vi "Invalid Text Color Write.vi"(4 "error in (no error)":errorcluster, 5 "Value":u32(colorbox)=8388608, 6 "Container State":T2, 7 "Display State In":T1={"format string"="%#_g", "font size"=13, "invalid text"="<Auto>", "valid range"={"min"=-inf, "max"=0.0}, "size"={"width"=100, "height"=22}, "numeric text color"=0, "overlay text color"=6553600}) -> (0 "error out":errorcluster, 3 "Display State Out":T1={"format string"="%#_g", "font size"=13, "invalid text"="<Auto>", "valid range"={"min"=-inf, "max"=0.0}, "size"={"width"=100, "height"=22}, "numeric text color"=0, "overlay text color"=6553600})   [LabVIEW 2017, in "Numeric with String Overlay.xctl"]
uses:
  <vilib>/addons/_XControls/Numeric with String Overlay/Numeric with String Overlay.xctl
  <vilib>/_xctls/Container State.ctl
  <vilib>/addons/_XControls/Numeric with String Overlay/State.ctl
  <vilib>/_xctls/XControlSupport.lvlib
panel:
  # "Replace the Value Control below with a Control of desired type.\nDo not remove this Control or the others from the connector pane.\nDo not change the connector pane pattern.\nThe Value control should always be the third terminal from top on the input side in the connector pane."
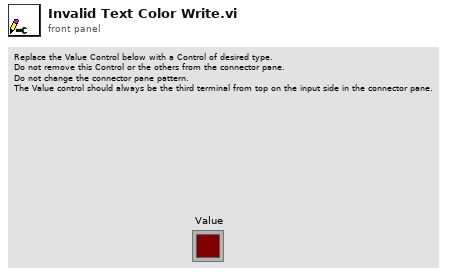
[diagram p1: front panel]
types:
  T1 = typedef "Numeric with String Overlay.xctl/State.ctl" = cluster{"format string":string, "font size":u32, "invalid text":string, "valid range":cluster{"min":dbl, "max":dbl}, "size":cluster{"width":u32, "height":u32}, "numeric text color":u32, "overlay text color":u32}
  T2 = typedef "XControlSupport.lvlib/Container State.ctl" = cluster{"Indicator?":bool, "Run Mode?":bool, " Refnum":refnum<vi>}
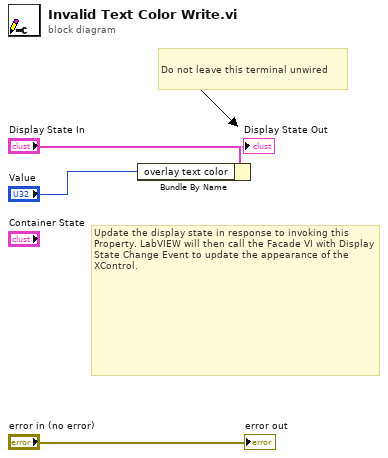
[diagram p0: block diagram]
diagram:
  # "Do not leave this terminal unwired"
  # "Update the display state in response to invoking this Property. LabVIEW will then call the Facade VI with Display State Change Event to update the appearance of the XControl."
  n1 = Bundle By Name(cluster="Display State In", "overlay text color"="Value") -> (→"Display State Out":T1)
  "error out" <- "error in (no error)"
